vi "Read Outputs to system.vi"(8 "error in":errorcluster, 11 "ScaleAndLimitModule runtime in":refnum<class "ScaleAndLimitModule runtime.lvclass">) -> (0 "error out":errorcluster, 2 "Outputs to system":T1, 3 "ScaleAndLimitModule runtime out":refnum<class "ScaleAndLimitModule runtime.lvclass">)   [LabVIEW 2017, in "ScaleAndLimitModule runtime.lvclass"]
uses:
  ScaleAndLimitModule runtime.lvclass
  configuration/output data indices.ctl
  ScaleAndLimitModule runtime.lvclass/ScaleAndLimitModule runtime.ctl
  configuration/ScaleAndLimitModule configuration.lvclass
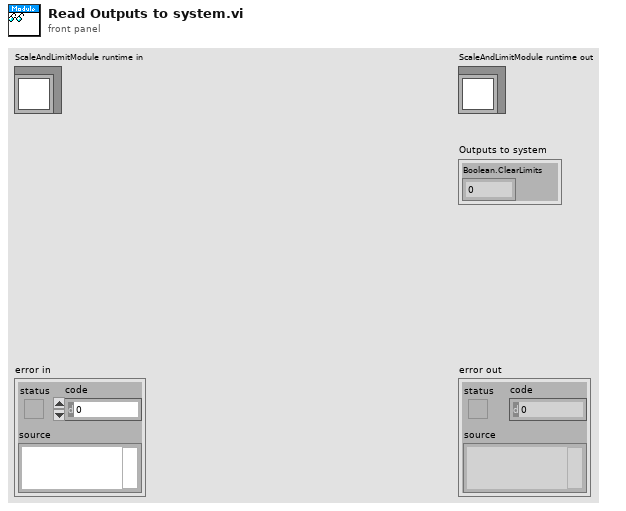
[diagram p1: front panel]
types:
  T1 = typedef "ScaleAndLimitModule configuration.lvclass/output data indices.ctl" = cluster{"Boolean.ClearLimits":i32}
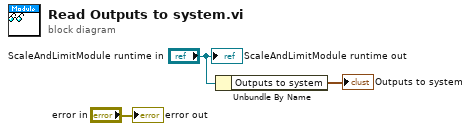
[diagram p0: block diagram]
diagram:
  n1 = Unbundle By Name("ScaleAndLimitModule runtime in") -> ("Outputs to system"=→"Outputs to system":T1)
  "error out" <- "error in"
  "ScaleAndLimitModule runtime out" <- "ScaleAndLimitModule runtime in"
